vi "test2-StateChange_Queue.vi"(8 "error in (no error)":errorcluster, 11 "TestCase in":refnum<class "testcase-CSMGlobalLog.lvclass">) -> (0 "error out":errorcluster, 3 "TestCase out":refnum<class "testcase-CSMGlobalLog.lvclass">)   [LabVIEW 2017, in "testcase-CSMGlobalLog.lvclass"]
uses:
  testcase-CSMGlobalLog.lvclass
  testcase-CSMGlobalLog.lvclass/testcase-CSMGlobalLog.ctl
  650155f4-1af1-443b-a877-8bdf29044e93.vi
  <vilib>/addons/_JKI Toolkits/VI Tester/TestCase.llb/TestCase.lvclass
  src/user.lib/_NEVSTOP/Communicable State Machine(CSM)/Utility/Periodic String Filter Setting.ctl
  src/user.lib/_NEVSTOP/Communicable State Machine(CSM)/Communicable State Machine.lvlib
  CSM/CSM-Testcase.lvlib
  C:/Program Files (x86)/National Instruments/LabVIEW 2017/vi.lib/addons/_JKI Toolkits/VI Tester/TestCase.llb/TestCase.lvclass
panel:
  out "String cache total":string
  out "LoopCount":i32
  out "String Cache Each Loop":string
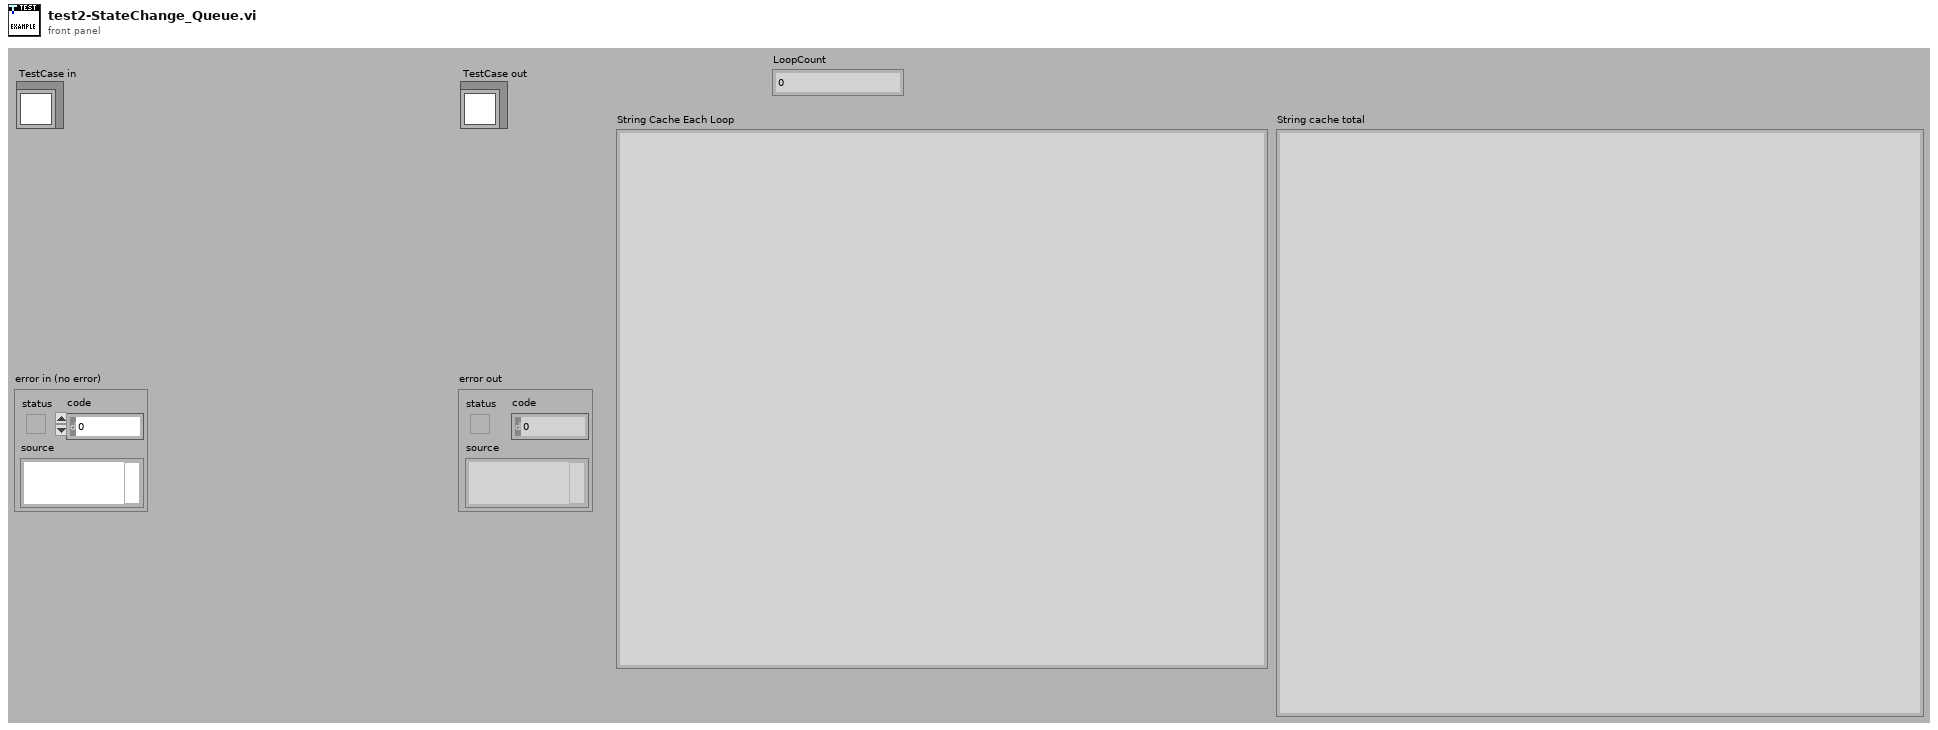
[diagram p1: front panel]
types:
  T1 = typedef "Communicable State Machine.lvlib/Periodic String Filter Setting.ctl" = cluster{"threashold(#/s)":dbl, "Check Peroid(s)":dbl}
  T2 = typedef "Communicable State Machine.lvlib/_CSM_GlobalLog_MSG.ctl" = cluster{"Name (\"\" to Use UUID)":string, "Current State":string, "Arguments":string, "Source Message":T3, "Source Module":string, "Complete(T)/Start(F)":bool, "LogType":T4, "Time Stamp":timestamp}
  T3 = typedef "Communicable State Machine.lvlib/_CSM_Response Source Message.ctl" = cluster{"‘State":string, "’Arguments":string, "’Error":errorcluster}
  T4 = typedef "Communicable State Machine.lvlib/_CSM_GlobalLog_MSG_TYPE.ctl" = enum16{"User Log", "State Change", "Status", "Interrupt", "Register", "Unregister", "Error Log", "Module Created", "Module Destroyed", "Async Message", "No-Rep Async Message", "Sync Message"}
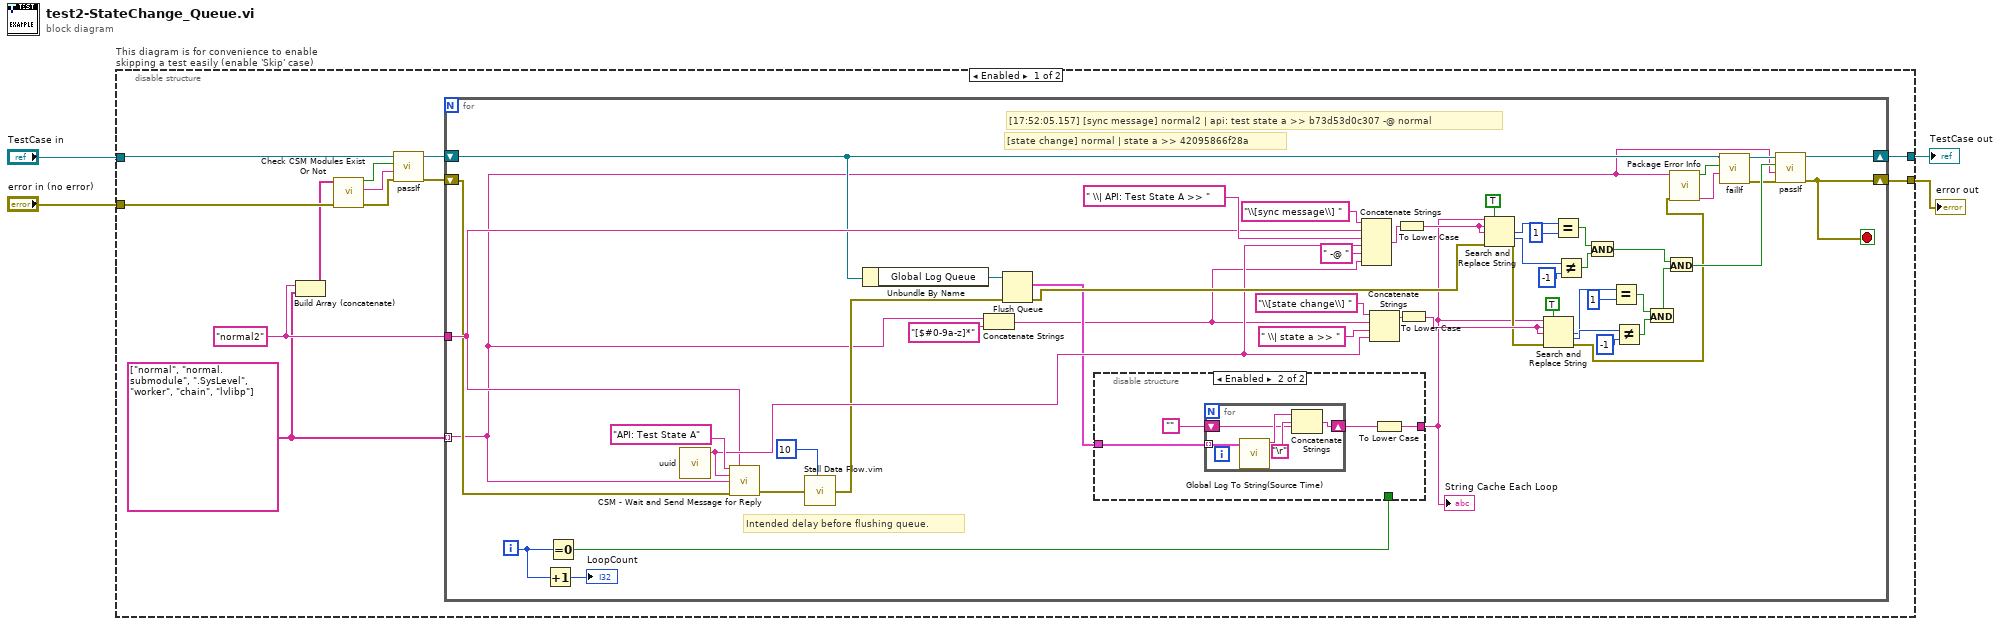
[diagram p0: block diagram]
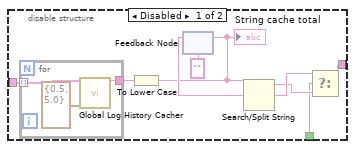
[diagram p2: hidden frame]
diagram:
  n1 = disable-structure "This diagram is for convenience to enable skipping a test easily (enable 'Skip' case)" shown="Enabled" {
    disable-tunnel: "TestCase in" -> [w11 w93]
    disable-tunnel: [w15 w91] -> w1
    disable-tunnel: [w16 w92] -> w3
    disable-tunnel: "error in (no error)" -> [w8 w90]
    frame Enabled {
      w7 = "normal2" ("CSM")
      w6 = string[] ["normal", "normal.submodule", ".SysLevel", "worker", "chain", "lvlibp"]
      n2 = Build Array (concatenate)(w7, w6) -> (w5:string[])
      n3 = call "Check CSM Modules Exist Or Not.vi"("error in"=w8, "CSM names in"=w5) -> ("error out"=w12:errorcluster, "Debug string"=w13:string, "All Modules Exist?"=w14:bool)  [unwired: 7 in]
      n4 = call-dynamic "passIf.vi"("error in (no error)"=w12, "message (\"\")"=w13, "pass"=w14, "TestCase in"=w11) -> ("error out"=w9:errorcluster, "TestCase out"=w10:refnum<class "testcase-CSMGlobalLog.lvclass">)  [unwired: 6 in]
      n5 = for {
        tunnel: w6 -> [w17] mode=indexing
        shift-right: [w36] -> w16
        shift-left: w9 -> [w24]
        shift-right: [w68] -> w15
        shift-left: w10 -> [w19]
        tunnel: w7 -> [w26]
        i -> [w28]
        stop <- w36 stop-if-true
        # "[17:52:05.157] [sync message] normal2 | api: test state a >> b73d53d0c307 -@ normal"
        # "Intended delay before flushing queue."
        # "[state change] normal | state a >> 42095866f28a"
        n6 = Increment(x=w28) -> (x+1=→"LoopCount":i32)
        n7 = Equal To 0?(x=w28) -> (x = 0?=w27:bool)
        n8 = call "uuid.vi"() -> ("UUID"=w39:string)  [unwired: 11 in]
        n9 = call "CSM - Wait and Send Message for Reply.vi"("State"="API: Test State A", "Current Module (\"\" to Generate an ID)"=w26, "Arguments (\"\")"=w39, "Target Module"=w17, "Error In (No Error)"=w24) -> ("error out"=w33:errorcluster)  [unwired: 7 in, 3 out]
        n10 = call "Stall Data Flow.vim"("value in"=w33, "milliseconds to wait"=u32 10) -> ("value out"=w32:errorcluster)  [unwired: 1 out]
        n11 = Unbundle By Name(w19) -> ("Global Log Queue"=w67:refnum<queue>)
        n12 = Concatenate Strings(w17, "[$#0-9a-z]*" ("string")) -> (w25:string)
        n13 = Flush Queue(queue=w67, error in (no error)=w32) -> (remaining elements=w30:T2[], error out=w45:errorcluster)  [unwired: 1 out]
        n14 = disable-structure shown="Enabled" {
          disable-tunnel: [w71 w81] -> w29
          disable-tunnel: w27 -> [w70 _]
          disable-tunnel: w30 -> [w69 w83]
          frame Disabled {
            n15 = for {
              tunnel: w69 -> [w80] mode=indexing
              tunnel: [w79] -> w77
              n16 = call "Global Log History Cacher.vi"("Global Log Data"=w80, "Settings"=T1 {"threashold(#/s)"=0.5, "Check Peroid(s)"=5.0}) -> ("String Cache"=w79:string)  [unwired: 13 in]
            }
            n17 = To Lower Case(string=w77) -> (all lower case string=w72:string)
            "String cache total" <- w72
            n18 = feedback #1("") -> (w76:string)
            n19 = feedback-in #1(w72) -> ()
            n20 = Search/Split String(string=w72, search string/char (-)=w76) -> (substring before match=w73:string, match + rest of string=w74:string)  [unwired: 1 in, 1 out]
            n21 = Select(t=w74, s=w70, f=w73) -> (s? t:f=w71:string)
          }
          frame Enabled {
            n22 = for {
              tunnel: w83 -> [w89] mode=indexing
              shift-right: [w85] -> w82
              shift-left: "" -> [w86]
              n23 = call "Global Log To String(Source Time).vi"("Log"=w89) -> ("Log String"=w88:string)  [unwired: 9 in]
              n24 = Concatenate Strings(w88, "\r", w86) -> (w85:string)
            }
            n25 = To Lower Case(string=w82) -> (all lower case string=w81:string)
          }
        }
        "String Cache Each Loop" <- w29
        n26 = Concatenate Strings("\\[sync message\\] " ("regular expression"), w26, " \\| API: Test State A >> " ("string"), w39, " -@ " ("string"), w25) -> (w62:string)
        n27 = Concatenate Strings("\\[state change\\] " ("regular expression"), w25, " \\| state a >> " ("string"), w39) -> (w64:string)
        n28 = To Lower Case(string=w62) -> (all lower case string=w60:string)
        n29 = To Lower Case(string=w64) -> (all lower case string=w48:string)
        n30 = Search and Replace String(replace all?=TRUE ("replace all? (F)"), input string=w29, search string=w60, replace string=w60, error in=w45) -> (number of replacements=w59:i32, offset past replacement=w58:i32, error out=w47:errorcluster)  [unwired: 3 in, 1 out]
        n31 = Search and Replace String(replace all?=TRUE ("replace all? (F)"), input string=w29, search string=w48, replace string=w48, error in=w47) -> (number of replacements=w50:i32, offset past replacement=w51:i32, error out=w18:errorcluster)  [unwired: 3 in, 1 out]
        n32 = Equal?(x=w59, y=1) -> (x = y?=w56:bool)
        n33 = Not Equal?(x=w58, y=-1) -> (x != y?=w55:bool)
        n34 = And(x=w56, y=w55) -> (x .and. y?=w37:bool)
        n35 = Equal?(x=w50, y=1) -> (x = y?=w53:bool)
        n36 = Not Equal?(x=w51, y=-1) -> (x != y?=w54:bool)
        n37 = And(x=w53, y=w54) -> (x .and. y?=w46:bool)
        n38 = And(x=w37, y=w46) -> (x .and. y?=w34:bool)
        n39 = call "Package Error Info.vi"("error in"=w18, "String in"=w17) -> ("packed error info out"=w22:string, "error status"=w23:bool)  [unwired: 8 in]
        n40 = call-dynamic "failIf.vi"("message (\"\")"=w22, "fail"=w23, "TestCase in"=w19) -> ("error out"=w20:errorcluster, "TestCase out"=w21:refnum<class "testcase-CSMGlobalLog.lvclass">)  [unwired: 7 in]
        n41 = call-dynamic "passIf.vi"("error in (no error)"=w20, "message (\"\")"=w17, "pass"=w34, "TestCase in"=w21) -> ("error out"=w36:errorcluster, "TestCase out"=w68:refnum<class "testcase-CSMGlobalLog.lvclass">)  [unwired: 6 in]
      }
    }
    frame Disabled {
      # "skip test result while test is under development"
      n42 = call <vilib>:"skip.vi"("error in (no error)"=w90, "TestCase in"=w93) -> ("error out"=w92:errorcluster, "TestCase out"=w91:refnum<class "testcase-CSMGlobalLog.lvclass">)  [unwired: 8 in]
    }
  }
  "error out" <- w3
  "TestCase out" <- w1
